vi "Func_AddToPolymorph.vi"(8 "error in (no error)":errorcluster, 9 "Name":string, 10 "New VI's Path":path, 11 "Polymorphic VI Path":path) -> (0 "error out":errorcluster, 4 "Polymorph count":i32)   [LabVIEW 2010, in "TemplateGenerator.lvlib"]
uses:
  TemplateGenerator.lvlib
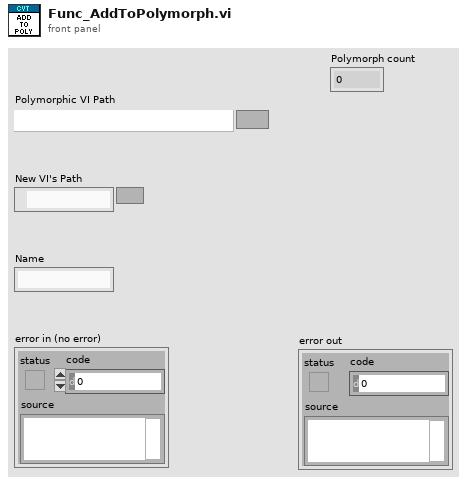
[diagram p1: front panel]
types:
  T1 = cluster{"VIPath":path, "Menu Name":string, "Selector Name":string}
  T2 = cluster{"VIPath":path, "Menu Name":string, "Selector Name":string}[]
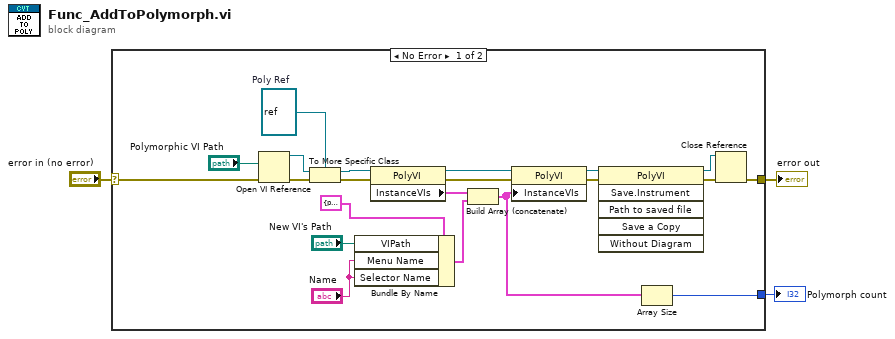
[diagram p0: block diagram]
diagram:
  n1 = case shown="No Error" "error in (no error)" {
    selector: "error in (no error)" -> [w6 w25]
    tunnel: [w16 w25] -> w3
    tunnel: [w4 _] -> w1
    frame No Error {
      w7 = refnum<vi> refnum  # Poly Ref
      n2 = Open VI Reference(vi path="Polymorphic VI Path", error in (no error)=w6) -> (vi reference=w9:refnum<vi>, error out=w22:errorcluster)  [unwired: 4 in]
      n3 = To More Specific Class(target class=w7, reference=w9, error in=w22) -> (specific class reference=w8:refnum<vi>, error out=w10:errorcluster)
      n4 = Bundle By Name(cluster=T1 {"VIPath"=path "", "Menu Name"="", "Selector Name"=""}, "VIPath"="New VI's Path", "Menu Name"="Name", "Selector Name"="Name") -> (w13:T1)
      n5 = property class="PolyVI"(reference=w8, error in=w10) -> (reference out=w21:refnum<vi>, error out=w20:errorcluster, "InstanceVIs"=w15:T2)
      n6 = Build Array (concatenate)(w15, w13) -> (w5:T2)
      n7 = property class="PolyVI"(reference=w21, error in=w20, "InstanceVIs"=w5) -> (reference out=w18:refnum<vi>, error out=w19:errorcluster)
      n8 = invoke class="PolyVI" method="Save.Instrument"(reference=w18, error in=w19) -> (reference out=w23:refnum<vi>, error out=w24:errorcluster)  [unwired: 4 in, 4 out]
      n9 = Array Size(array=w5) -> (size(s)=w4:i32)
      n10 = Close Reference(reference=w23, error in (no error)=w24) -> (error out=w16:errorcluster)
    }
    frame Error {
    }
  }
  "error out" <- w3
  "Polymorph count" <- w1
